vi "getOutllookPaths.vi"(8 "error in (no error)":errorcluster, 11 "reference in":refnum<class "File Controller.lvclass">) -> (0 "error out":errorcluster, 3 "reference out":refnum<class "File Controller.lvclass">)   [LabVIEW 2014, in "File Controller.lvclass"]
uses:
  File Controller.lvclass
  <vilib>/Utility/config.llb/Read Key (Path).vi
  <vilib>/Utility/config.llb/NI_LVConfig.lvlib
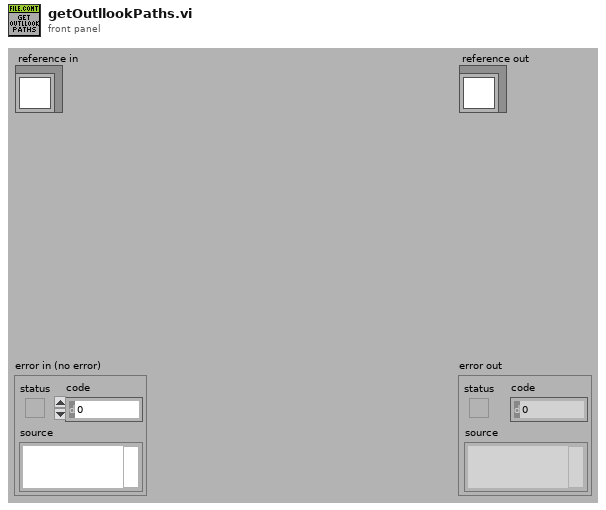
[diagram p1: front panel]
types:
  T1 = typedef "File Controller.lvclass/ObjectAttributesRef.ctl" = refnum<data-value>
  T2 = typedef "File Controller.lvclass/ObjectAttributes.ctl" = cluster{"MyAttribute":dbl, "excelFile_refs":refnum<class "excelFile.lvclass">[], "filePaths":path[], "outlookTemplatePaths":path[], "attachmentTemplatePaths":path[], "configFilePath":path, "not_setting":bool[], "python_ref":refnum<class "python.lvclass">}
  T3 = typedef "NI_LVConfig.lvlib/Config Data RefNum.ctl" = refnum<k1>
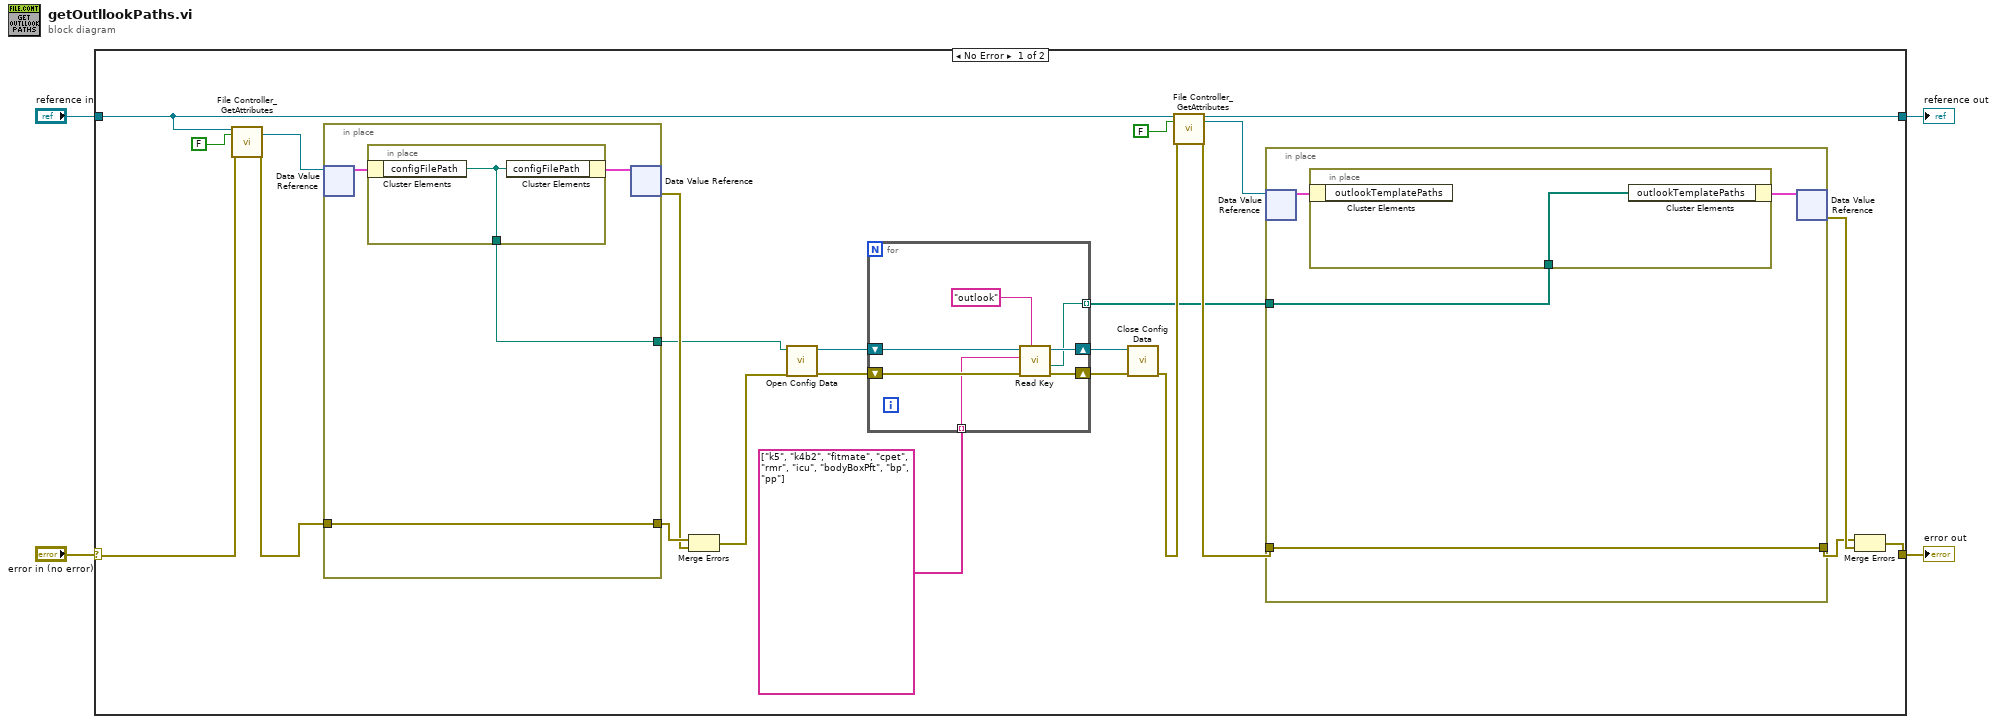
[diagram p0: block diagram]
diagram:
  n1 = case shown="No Error" "error in (no error)" {
    selector: "error in (no error)" -> [w9 w46]
    tunnel: [w27 w46] -> w3
    tunnel: [w22 w45] -> w1
    tunnel: "reference in" -> [w8 w45]
    frame No Error {
      n2 = call "File Controller_GetAttributes.vi"("reference in"=w8, "return data? (T)"=FALSE, "error in (no error)"=w9) -> ("attributes ref"=w13:T1, "error out"=w7:errorcluster)  [unwired: 13 in, 2 out]
      n3 = in-place {
        in-place-border: w7 -> [w29]
        in-place-border: [w29] -> w11
        in-place-border: [w28] -> w5
        n4 = in-place-dvr #1(w13) -> (w30:T2)  [unwired: 1 out]
        n5 = in-place {
          in-place-border: [w32] -> w28
          n6 = in-place-cluster #2(w30) -> ("configFilePath"=w32:path)
          n7 = in-place-cluster #2("configFilePath"=w32) -> (w31:T2)
        }
        n8 = in-place-dvr #1(w31) -> (w10:errorcluster)  [unwired: 1 out]
      }
      n9 = Merge Errors(w11, w10) -> (w6:errorcluster)
      n10 = call <vilib>:"Open Config Data.vi"("error in (no error)"=w6, "configuration file path"=w5) -> ("error out"=w19:errorcluster, "refnum"=w20:T3)  [unwired: 7 in, 1 out]
      n11 = for {
        shift-right: [w36] -> w18
        shift-left: w20 -> [w39]
        shift-right: [w35] -> w17
        shift-left: w19 -> [w38]
        tunnel: string[] ["k5", "k4b2", "fitmate", "cpet", "rmr", "icu", "bodyBoxPft", "bp", "pp"] -> [w34] mode=indexing
        tunnel: [w33] -> w14 mode=indexing
        n12 = call-poly <vilib>:"Read Key.vi"("section"="outlook", "error in (no error)"=w38, "key"=w34, "refnum"=w39) -> ("error out"=w35:errorcluster, "value"=w33:path, "refnum out"=w36:T3)  [unwired: 4 in, 1 out]
      }
      n13 = call <vilib>:"Close Config Data.vi"("error in (no error)"=w17, "refnum"=w18) -> ("error out"=w15:errorcluster)  [unwired: 8 in, 1 out]
      n14 = call "File Controller_GetAttributes.vi"("reference in"=w8, "return data? (T)"=FALSE, "error in (no error)"=w15) -> ("reference out"=w22:refnum<class "File Controller.lvclass">, "attributes ref"=w21:T1, "error out"=w23:errorcluster)  [unwired: 13 in, 1 out]
      n15 = in-place {
        in-place-border: w23 -> [w41]
        in-place-border: [w41] -> w25
        in-place-border: w14 -> [w40]
        n16 = in-place-dvr #3(w21) -> (w42:T2)  [unwired: 1 out]
        n17 = in-place {
          in-place-border: w40 -> [w44]
          n18 = in-place-cluster #4(w42) -> ()  [unwired: 1 out]
          n19 = in-place-cluster #4("outlookTemplatePaths"=w44) -> (w43:T2)
        }
        n20 = in-place-dvr #3(w43) -> (w26:errorcluster)  [unwired: 1 out]
      }
      n21 = Merge Errors(w25, w26) -> (w27:errorcluster)
    }
    frame Error {
    }
  }
  "error out" <- w3
  "reference out" <- w1
